vi "New.vi"(0 "Topic":string, 5 "Notify result":bool, 7 "Arguments":string, 9 "ArgumentsKw":string="{}", 11 "error in (no error)":errorcluster, 12 "Options":string="{}") -> (4 "Publish JSON out":refnum<class "Publish JSON.lvclass">, 6 "Notifier out":refnum<notifier>, 15 "error out":errorcluster)   [LabVIEW 2020, in "wamplv.lvlib" / "Publish JSON.lvclass"]
uses:
  Publish JSON.lvclass
  Publish JSON.lvclass/Publish JSON.ctl
  ef80e5bd-c3b5-48bf-80d2-81f5adeaff0a.vi
  Message loop classes/ErrorOrSuccess JSON/ErrorOrSuccess JSON.lvclass
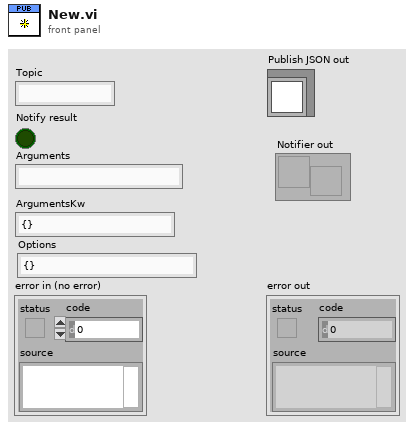
[diagram p1: front panel]
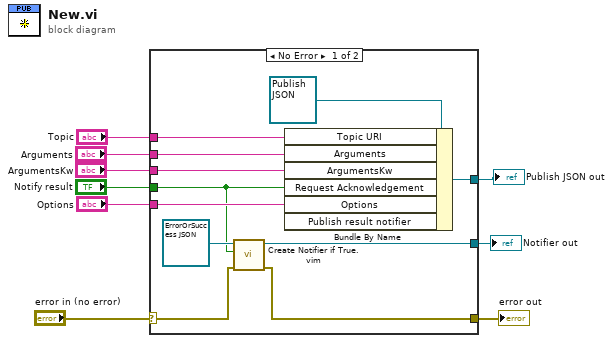
[diagram p0: block diagram]
diagram:
  n1 = case shown="No Error" "error in (no error)" {
    selector: "error in (no error)" -> [w13 w21]
    tunnel: [w12 w21] -> w8
    tunnel: "Topic" -> [w19 _]
    tunnel: "Arguments" -> [w18 _]
    tunnel: "ArgumentsKw" -> [w17 _]
    tunnel: "Notify result" -> [w14 _]
    tunnel: "Options" -> [w16 _]
    tunnel: [w11 _] -> w2
    tunnel: [w10 _] -> w1
    frame No Error {
      n2 = call "Create Notifier if True.vim"("error in (no error)"=w13, "Boolean"=w14, "RESULT Payload"=refnum<class "ErrorOrSuccess JSON.lvclass"> refnum ("wamplv.lvlib:ErrorOrSuccess JSON.lvclass")) -> ("error out"=w12:errorcluster, "Notifier out"=w10:refnum<notifier>)  [unwired: 7 in]
      n3 = Bundle By Name(cluster=refnum<class "Publish JSON.lvclass"> refnum ("wamplv.lvlib:Publish JSON.lvclass"), "Topic URI"=w19, "Arguments"=w18, "ArgumentsKw"=w17, "Request Acknowledgement"=w14, "Options"=w16) -> (w11:refnum<class "Publish JSON.lvclass">)  [unwired: 1 in]
    }
    frame Error {
    }
  }
  "error out" <- w8
  "Publish JSON out" <- w2
  "Notifier out" <- w1
